vi "VI.vi"() -> ()   [LabVIEW 2014]
uses:
  <vilib>/Platform/TimedLoop/XDataNode/timing_clust.ctl
  <vilib>/Platform/TimedLoop/XDataNode/nitl_modes.ctl
  <vilib>/Platform/TimedLoop/XDataNode/wakeup.ctl
  <vilib>/platform/TimedLoop/XDataNode/XDataNode.xnode
  <vilib>/Platform/TimedLoop/XDataNode/XDNodeRunTimeDep.lvlib
panel:
  in  "base size":i32=100000
  in  "count":i32=2
  out "dt":dbl=0.164769041351974
  out "element":dbl=0.4179459052036547
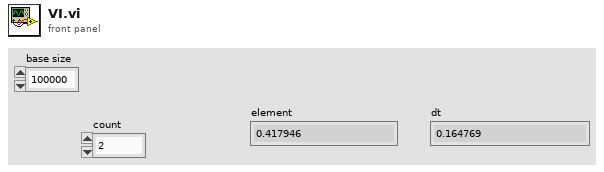
[diagram p1: front panel]
types:
  T1 = typedef "XDNodeRunTimeDep.lvlib/timing_clust.ctl" = cluster{"Expected End [f-1]":u64, "Actual End [f-1]":u64, "Finished Late? [f-1]":bool, "Expected End [i-1]":u64, "Actual End [i-1]":u64, "Finished Late? [i-1]":bool, "Expected Start [i]":u64, "Actual Start [i]":u64, "Expected Start [f]":u64, "Actual Start [f]":u64, "Source Name":string, "Structure Name":string, "Period":i64, "Deadline":i64, "Offset":i64, "Start":i64, "Priority":i32, "Timeout":i32, "Mode":T2, "Wakeup Reason":T3, "Error":errorcluster, "Source Type":string, "Secondary Source Type":string, "Global End Time":u64, "Global Start Time":u64, "Frame Duration":u64, "Iteration Duration":u64, "Assigned CPU":i32, "I/O Scan Engine Mode":u32}
  T2 = typedef "XDNodeRunTimeDep.lvlib/nitl_modes.ctl" = enum32{"No Change", "Process missed periods, maintain original phase", "Discard missed periods, maintain original phase", "Process missed periods, ignore original phase", "Discard missed periods, ignore original phase"}
  T3 = typedef "XDNodeRunTimeDep.lvlib/wakeup.ctl" = enum32{"Normal", "Aborted", "Asynchronous wakeup", "Timing source error", "Timed loop error", "Timeout"}
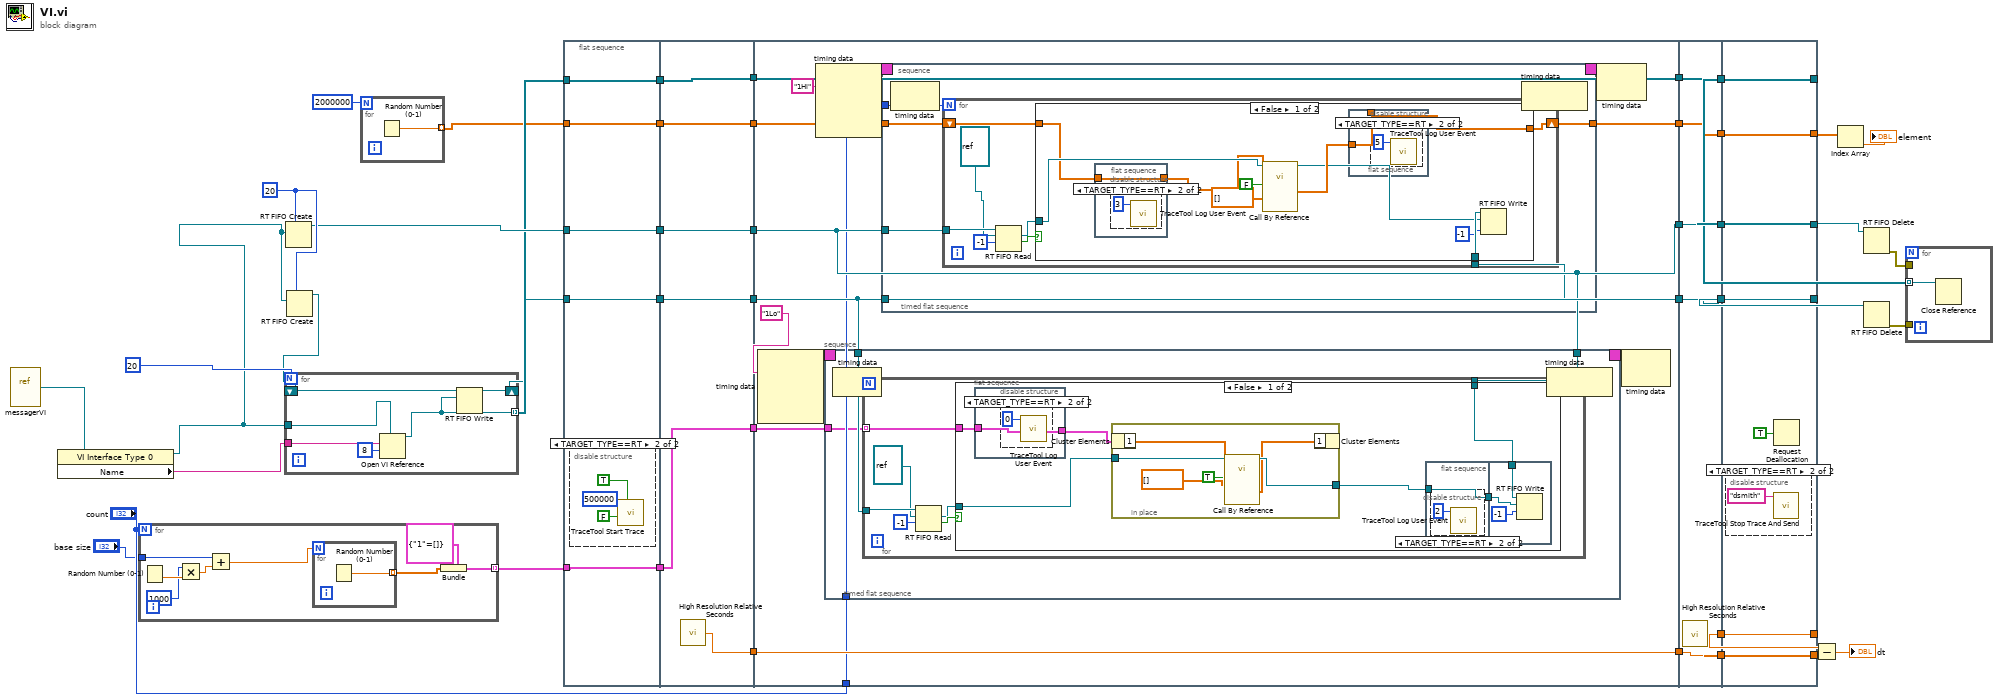
[diagram p0: block diagram]
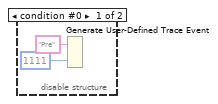
[diagram p2: hidden frame]
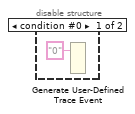
[diagram p3: hidden frame]
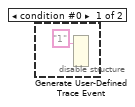
[diagram p4: hidden frame]
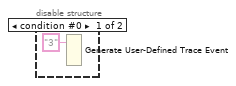
[diagram p6: hidden frame]
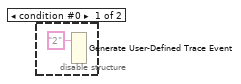
[diagram p7: hidden frame]
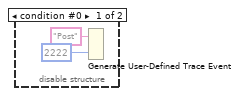
[diagram p9: hidden frame]
diagram:
  w46 = u32 20 ("size (10)")
  n1 = vi-ref "messagerVI.vi"() -> (w4:refnum<vi>)
  n2 = property class="VI Interface Type 0"(reference=w4) -> (reference out=w2:refnum<vi>, "Name"=w3:string)  [unwired: 1 in, 1 out]
  n3 = for {
    N: "count" -> [_]
    tunnel: [w53] -> w44 mode=indexing
    tunnel: "base size" -> [w47]
    n4 = Random Number (0-1)() -> (number: 0 to 1=w52:dbl)
    n5 = Multiply(x=1000, y=w52) -> (x*y=w51:dbl)
    n6 = Add(x=w47, y=w51) -> (x+y=w49:dbl)
    n7 = for {
      N: w49 -> [_]
      tunnel: [w55] -> w54 mode=indexing
      n8 = Random Number (0-1)() -> (number: 0 to 1=w55:dbl)
    }
    n9 = Bundle(cluster=cluster{"1":dbl[]} {"1"=[]}, "1"=w54) -> (w53:cluster{"1":dbl[]})
  }
  n10 = RT FIFO Create(1:w2, 4:w46) -> (8:w43:refnum<k33>)  [unwired: 6 in, 2 out]
  n11 = RT FIFO Create(1:w2, 4:w46) -> (8:w26:refnum<k33>)  [unwired: 6 in, 2 out]
  n12 = for {
    N: 20 -> [_]
    tunnel: [w58] -> w36 mode=indexing
    shift-right: [w60] -> w25
    shift-left: w26 -> [w61]
    tunnel: w3 -> [w59]
    tunnel: w2 -> [w56]
    n13 = Open VI Reference(type specifier VI Refnum (for type only)=w56, vi path=w59, options=8) -> (vi reference=w58:refnum<vi>)  [unwired: 3 in, 1 out]
    n14 = RT FIFO Write(0:w61, 1:w58) -> (8:w60:refnum<k33>)  [unwired: 3 in, 3 out]
  }
  n15 = for {
    N: 2000000 -> [_]
    tunnel: [w62] -> w22 mode=indexing
    n16 = Random Number (0-1)() -> (number: 0 to 1=w62:dbl)
  }
  n17 = flat-sequence {
    tunnel: w22 -> [w63]
    tunnel: w36 -> [w64]
    tunnel: w43 -> [w65]
    tunnel: w25 -> [w66]
    tunnel: w44 -> [w67]
    tunnel: [w67] -> w9
    tunnel: [w66] -> w8
    tunnel: [w65] -> w7
    tunnel: [w64] -> w6
    tunnel: [w63] -> w5
    tunnel: [w78] -> w41
    tunnel: [w77] -> w39
    tunnel: [w76] -> w35
    tunnel: [w75] -> w29
    tunnel: [w74] -> w23
    tunnel: [w73] -> w17
    tunnel: w9 -> [w73]
    tunnel: w8 -> [w77]
    tunnel: w7 -> [w78]
    tunnel: w6 -> [w76]
    tunnel: w5 -> [w74]
    tunnel: [w87] -> w42
    tunnel: w41 -> [w87]
    tunnel: [w88] -> w40
    tunnel: w39 -> [w88]
    tunnel: w35 -> [w92]
    tunnel: [w92] -> w34
    tunnel: w29 -> [w91]
    tunnel: [w91] -> w28
    tunnel: w23 -> [w90]
    tunnel: [w89] -> w21
    tunnel: "count" -> [w86]
    tunnel: w17 -> [w85]
    tunnel: w42 -> [w181]
    tunnel: w40 -> [w180]
    tunnel: w34 -> [w179]
    tunnel: w28 -> [w177]
    tunnel: w21 -> [w176]
    tunnel: [w181] -> w15
    tunnel: [w180] -> w14
    tunnel: [w179] -> w13
    tunnel: [w178] -> w12
    tunnel: [w177] -> w11
    tunnel: [w176] -> w10
    tunnel: [w183] -> w20
    tunnel: [w184] -> w27
    tunnel: [w185] -> w30
    tunnel: [w186] -> w33
    tunnel: [w187] -> w37
    tunnel: [w188] -> w38
    tunnel: w15 -> [w188]
    tunnel: w14 -> [w187]
    tunnel: w13 -> [w186]
    tunnel: w12 -> [w185]
    tunnel: w11 -> [w184]
    tunnel: w10 -> [w183]
    frame #0 {
      n18 = disable-structure shown="TARGET_TYPE==RT" {
        frame condition #0 {
          n19 = Generate User-Defined Trace Event(1:1111 ("trace integer"), 2:"Pre" ("trace string")) -> ()
        }
        frame condition #1 (active) {
          n20 = call <vilib>:"TraceTool Start Trace.vi"("Detailed Tracing? (F)"=TRUE, "VI Tracing? (T)"=FALSE, "Buffer Size (250000 bytes)"=500000) -> ()  [unwired: 7 in, 2 out]
        }
      }
    }
    frame #1 {
      n21 = call <vilib>:"High Resolution Relative Seconds.vi"() -> ("relative seconds"=w75:dbl)
    }
    frame #2 {
      n22 = node-c288("1Lo" ("Structure Name")) -> (w82:T1)  [unwired: 3 in]
      n23 = node-c288("1Hi" ("Structure Name")) -> (w84:T1)  [unwired: 3 in]
      n24 = timed-sequence {
        timing: w82 -> [_]
        timing-out: [_] -> w81
        tunnel: w88 -> [w96]
        tunnel: w87 -> [w95]
        tunnel: w86 -> [w94]
        tunnel: w85 -> [w93]
        n25 = timed-flat-sequence {
          tunnel: w96 -> [w100]
          tunnel: w95 -> [w99]
          tunnel: w94 -> [w98]
          tunnel: w93 -> [w97]
          n26 = node-c288() -> ()  [unwired: 1 in, 1 out]
          n27 = for {
            N: w98 -> [_]
            tunnel: w100 -> [w107]
            tunnel: w99 -> [w103]
            tunnel: w97 -> [w102] mode=indexing
            n28 = RT FIFO Read(0:w107, 1:refnum<vi> refnum ("type specifier VI Refnum (for type only)"), 2:-1 ("timeout in ms (0)")) -> (9:w104:refnum<vi>, 10:w105:bool)  [unwired: 1 in, 3 out]
            n29 = case shown="False" w105 {
              tunnel: w104 -> [w110 _]
              tunnel: w103 -> [w113 _]
              tunnel: w102 -> [w112 _]
              frame False {
                n30 = flat-sequence {
                  tunnel: [w120] -> w108
                  tunnel: w112 -> [w120]
                  frame #0 {
                    n31 = disable-structure shown="TARGET_TYPE==RT" {
                      frame condition #0 {
                        n32 = Generate User-Defined Trace Event(2:"0" ("trace string")) -> ()  [unwired: 1 in]
                      }
                      frame condition #1 (active) {
                        n33 = call <vilib>:"TraceTool Log User Event.vi"("Event ID (0-255)"=u32 0) -> ()  [unwired: 10 in, 1 out]
                      }
                    }
                  }
                }
                n34 = in-place {
                  in-place-border: w110 -> [w119]
                  in-place-border: [w118] -> w109
                  n35 = in-place-cluster #1(w108) -> ("1"=w117:dbl[])
                  n36 = call-by-ref "?"(reference=w119, "msg data in"=w117, "data to change in"=dbl[] [] ("msg data in"), "T=Set, F=Act"=TRUE) -> (reference out=w118:refnum<vi>, "msg data out"=w116:dbl[])  [unwired: 8 in, 2 out]
                  n37 = in-place-cluster #1("1"=w116) -> ()  [unwired: 1 out]
                }
                n38 = flat-sequence {
                  tunnel: w109 -> [w123]
                  tunnel: [w123] -> w111
                  tunnel: w113 -> [w127]
                  tunnel: w111 -> [w126]
                  frame #0 {
                    n39 = disable-structure shown="TARGET_TYPE==RT" {
                      frame condition #0 {
                        n40 = Generate User-Defined Trace Event(2:"1" ("trace string")) -> ()  [unwired: 1 in]
                      }
                      frame condition #1 (active) {
                        n41 = call <vilib>:"TraceTool Log User Event.vi"("Event ID (0-255)"=u32 2) -> ()  [unwired: 10 in, 1 out]
                      }
                    }
                  }
                  frame #1 {
                    n42 = RT FIFO Write(0:w127, 1:w126, 2:-1 ("timeout in ms (0)")) -> ()  [unwired: 2 in, 4 out]
                  }
                }
              }
              frame True {
              }
            }
          }
          n43 = node-c288() -> ()  [unwired: 1 in, 1 out]
        }
      }
      n44 = timed-sequence {
        timing: w84 -> [_]
        timing-out: [_] -> w83
        tunnel: w90 -> [w139]
        tunnel: [w138] -> w89
        tunnel: w88 -> [w137]
        tunnel: w87 -> [w136]
        tunnel: w86 -> [w135]
        n45 = timed-flat-sequence {
          tunnel: w139 -> [w144]
          tunnel: [w143] -> w138
          tunnel: w137 -> [w142]
          tunnel: w136 -> [w141]
          tunnel: w135 -> [w140]
          n46 = node-c288() -> ()  [unwired: 1 in, 1 out]
          n47 = for {
            N: w140 -> [_]
            shift-right: [w149] -> w143
            shift-left: w144 -> [w148]
            tunnel: w141 -> [w152]
            tunnel: w142 -> [w146]
            n48 = RT FIFO Read(0:w152, 1:refnum<vi> refnum ("type specifier VI Refnum (for type only)"), 2:-1 ("timeout in ms (0)")) -> (9:w147:refnum<vi>, 10:w150:bool)  [unwired: 1 in, 3 out]
            n49 = case shown="False" w150 {
              tunnel: [w162 w169] -> w149
              tunnel: w148 -> [w155 w169]
              tunnel: w147 -> [w159 _]
              tunnel: w146 -> [w161 _]
              frame False {
                n50 = flat-sequence {
                  tunnel: [w166] -> w156
                  tunnel: w155 -> [w166]
                  frame #0 {
                    n51 = disable-structure shown="TARGET_TYPE==RT" {
                      frame condition #0 {
                        n52 = Generate User-Defined Trace Event(2:"2" ("trace string")) -> ()  [unwired: 1 in]
                      }
                      frame condition #1 (active) {
                        n53 = call <vilib>:"TraceTool Log User Event.vi"("Event ID (0-255)"=u32 3) -> ()  [unwired: 10 in, 1 out]
                      }
                    }
                  }
                }
                n54 = call-by-ref "?"(reference=w159, "msg data in"=dbl[] [], "data to change in"=w156, "T=Set, F=Act"=FALSE) -> (reference out=w154:refnum<vi>, "data to change out"=w157:dbl[])  [unwired: 8 in, 2 out]
                n55 = flat-sequence {
                  tunnel: [w163] -> w162
                  tunnel: w157 -> [w163]
                  frame #0 {
                    n56 = disable-structure shown="TARGET_TYPE==RT" {
                      frame condition #0 {
                        n57 = Generate User-Defined Trace Event(2:"3" ("trace string")) -> ()  [unwired: 1 in]
                      }
                      frame condition #1 (active) {
                        n58 = call <vilib>:"TraceTool Log User Event.vi"("Event ID (0-255)"=u32 5) -> ()  [unwired: 10 in, 1 out]
                      }
                    }
                  }
                }
                n59 = RT FIFO Write(0:w161, 1:w154, 2:-1 ("timeout in ms (0)")) -> ()  [unwired: 2 in, 4 out]
              }
              frame True {
              }
            }
          }
          n60 = node-c288() -> ()  [unwired: 1 in, 1 out]
        }
      }
      n61 = node-c288(w83) -> ()  [unwired: 1 out]
      n62 = node-c288(w81) -> ()  [unwired: 1 out]
    }
    frame #3 {
      n63 = call <vilib>:"High Resolution Relative Seconds.vi"() -> ("relative seconds"=w178:dbl)
    }
    frame #4 {
      n64 = disable-structure shown="TARGET_TYPE==RT" {
        frame condition #0 {
          n65 = Generate User-Defined Trace Event(1:2222 ("trace integer"), 2:"Post" ("trace string")) -> ()
        }
        frame condition #1 (active) {
          n66 = call <vilib>:"TraceTool Stop Trace And Send.vi"("Trace Host Network Address"="dsmith") -> ()  [unwired: 10 in, 1 out]
        }
      }
      n67 = Request Deallocation(TRUE ("flag")) -> ()
    }
  }
  n68 = Subtract(x=w30, y=w27) -> (x-y=→"dt":dbl)
  n69 = Index Array(array=w20) -> (element=→"element":dbl)  [unwired: 1 in]
  n70 = RT FIFO Delete(0:w38) -> (11:w31:errorcluster)  [unwired: 2 in]
  n71 = RT FIFO Delete(0:w37) -> (11:w32:errorcluster)  [unwired: 2 in]
  n72 = for {
    tunnel: w33 -> [w192] mode=indexing
    tunnel: w32 -> [_]
    tunnel: w31 -> [_]
    n73 = Close Reference(reference=w192) -> ()  [unwired: 1 in, 1 out]
  }
